vi "VMS_6_Controller.vi"() -> ()   [LabVIEW 2018]
uses:
  <vilib>/rvi/Emulation/niFpgaGetClockAttributes.vi
  <vilib>/rvi/Emulation/niFpgaSctlEmulationGetInTimedLoop.vi
  <vilib>/rvi/Emulation/niFpgaEmulationReportErrorSimple.vi
  <vilib>/rvi/Emulation/niFpgaProcessEmulError.vi
  <vilib>/rvi/eio/common/nirviEmuTemplateMethod_errors.vi
  <vilib>/rvi/Emulation/niFpgaCriticalErrorInLSC.vi
  <vilib>/rvi/interface/RandomDataEmulation/niFpgaRandomDataHandleErrors.vi
  <vilib>/rvi/occurrence/nirviWaitOnOccurrenceBase.vi
  <vilib>/eio/EIOMethodNode/EIOMethodNode.xnode
  <vilib>/rvi/DataTransferAndStorage/Container/XNode/niFpgaContainer.xnode
  <vilib>/rvi/interface/RandomDataEmulation/nirviRandomDataFpgaReadWriteTemplate.vi
  <vilib>/eio/EIONode/EIONode.xnode
panel:
  out "FIFO full":bool
  in  "Output type":i16
  in  "Period (ms)":u32=5
  out "Chassis Temperature":fxp<+/-,32,16>
  out "Stopped":bool
  out "Ready":bool
  out "Ticks":u64
  out "Timeouted":bool
  in  "Operate":bool
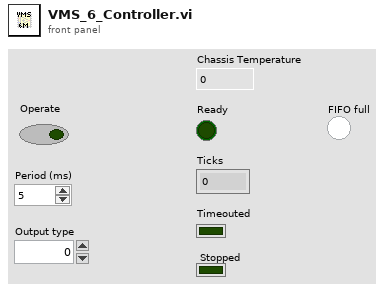
[diagram p1: front panel]
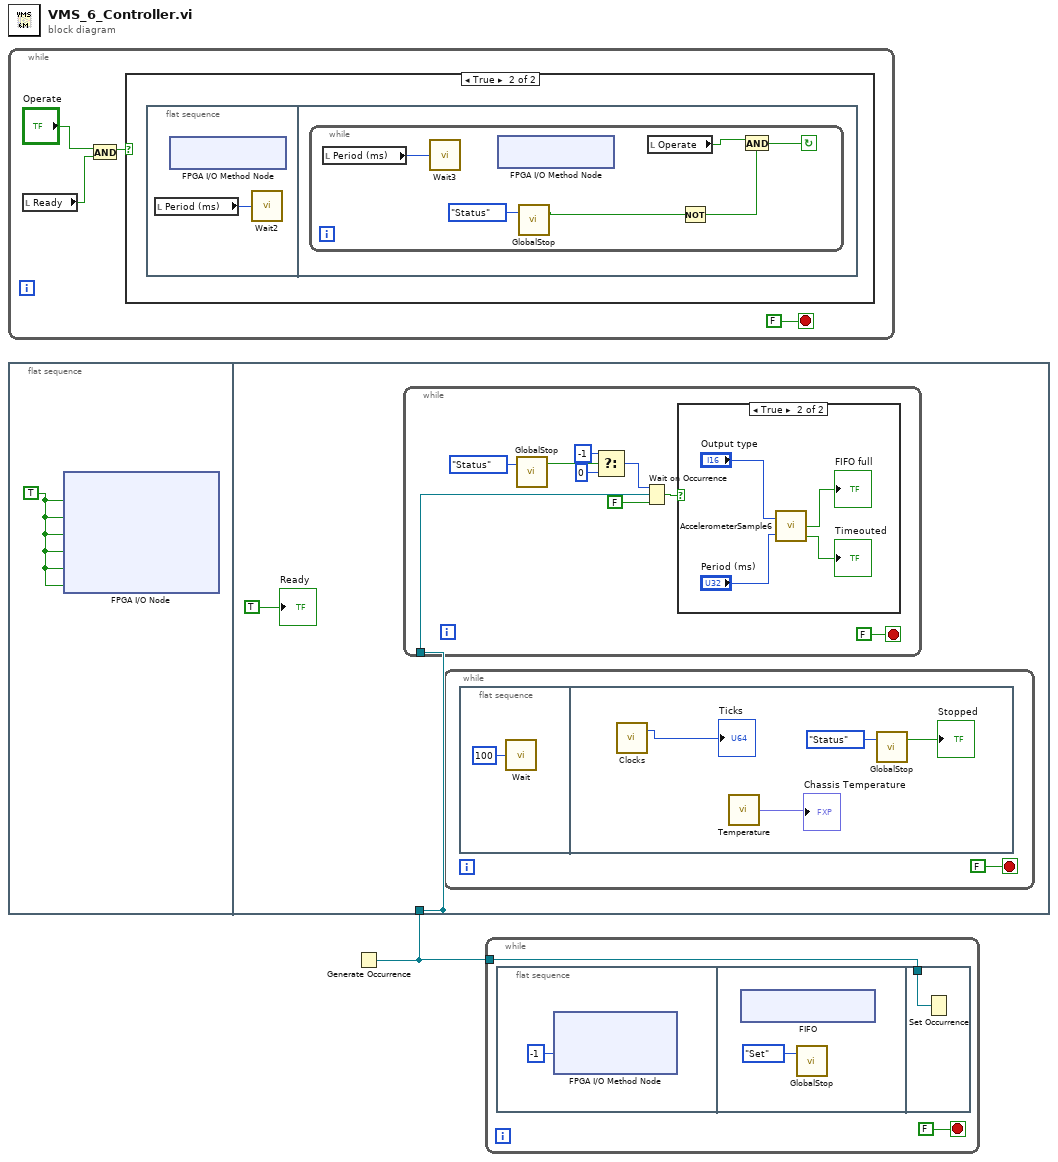
[diagram p0: block diagram]
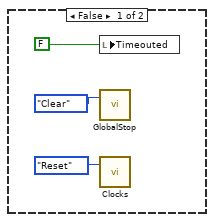
[diagram p2: hidden frame]
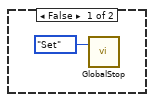
[diagram p3: hidden frame]
diagram:
  n1 = while {
    stop <- FALSE stop-if-true
    n2 = local read "Ready"() -> (w2:bool)
    n3 = And(x="Operate", y=w2) -> (x .and. y?=w4:bool)
    n4 = case shown="True" w4 {
      frame False {
        n5 = call "GlobalStop.vi"("Enum"=enum16{"Clear", "Set", "Status"}."Set") -> ()  [unwired: 1 in, 2 out]
      }
      frame True {
        n6 = flat-sequence {
          frame #0 {
            n7 = local read "Period (ms)"() -> (w7:u32)
            n8 = xnode "FPGA I/O Method Node"() -> ()  [unwired: 1 in, 1 out]
            n9 = call "Wait2"("Count(mSec)"=w7) -> ()  [unwired: 1 out]
          }
          frame #1 {
            n10 = while {
              stop <- w12 continue-if-true
              n11 = local read "Period (ms)"() -> (w8:u32)
              n12 = call "Wait3"("Count(mSec)"=w8) -> ()  [unwired: 1 out]
              n13 = xnode "FPGA I/O Method Node"() -> ()  [unwired: 1 in, 1 out]
              n14 = call "GlobalStop.vi"("Enum"=enum16{"Clear", "Set", "Status"}."Status") -> ("Boolean"=w9:bool)  [unwired: 1 in, 1 out]
              n15 = local read "Operate"() -> (w13:bool)
              n16 = Not(x=w9) -> (.not. x?=w11:bool)
              n17 = And(x=w13, y=w11) -> (x .and. y?=w12:bool)
            }
          }
        }
      }
    }
  }
  n18 = flat-sequence {
    tunnel: w1 -> [w15]
    tunnel: [w15] -> _
    frame #0 {
      w14 = TRUE ("Accelerometer5/Start")
      n19 = xnode "FPGA I/O Node"("Accelerometer1/Start"=w14, "Accelerometer2/Start"=w14, "Accelerometer3/Start"=w14, "Accelerometer4/Start"=w14, "Accelerometer5/Start"=w14, "Accelerometer6/Start"=w14) -> ()  [unwired: 6 in, 6 out]
    }
    frame #1 {
      n20 = while {
        tunnel: w15 -> [w28]
        stop <- FALSE stop-if-true
        n21 = call "GlobalStop.vi"("Enum"=enum16{"Clear", "Set", "Status"}."Status") -> ("Boolean"=w23:bool)  [unwired: 1 in, 1 out]
        n22 = Select(t=-1, s=w23, f=0) -> (s? t:f=w27:i32)
        n23 = Wait on Occurrence(1:FALSE ("ignore previous (T)"), 2:w28, 3:w27) -> (0:w29:bool)
        n24 = case shown="True" w29 {
          frame False {
            n25 = local write "Timeouted"(FALSE ("Timeouted")) -> ()
            n26 = call "GlobalStop.vi"("Enum"=enum16{"Clear", "Set", "Status"}."Clear") -> ()  [unwired: 1 in, 2 out]
            n27 = call "Clocks.vi"("Enum"=enum16{"Reset", "Increment", "Get"}."Reset") -> ()  [unwired: 1 in, 2 out]
          }
          frame True {
            n28 = call "AccelerometerSample6.vi"("Output type"="Output type", "Period (ms)"="Period (ms)") -> ("FIFO full"=→"FIFO full":bool, "Timeouted"=→"Timeouted":bool)  [unwired: 1 out]
          }
        }
      }
      n29 = while {
        stop <- FALSE stop-if-true
        n30 = flat-sequence {
          frame #0 {
            n31 = call "Wait"("Count(mSec)"=u32 100) -> ()  [unwired: 1 out]
          }
          frame #1 {
            n32 = call "Clocks.vi"() -> ("Clock"=→"Ticks":u64)  [unwired: 2 in, 1 out]
            n33 = call "Temperature.vi"() -> ("Mean temperature"=→"Chassis Temperature":fxp<+/-,32,16>)  [unwired: 1 in]
            n34 = call "GlobalStop.vi"("Enum"=enum16{"Clear", "Set", "Status"}."Status") -> ("Boolean"=→"Stopped":bool)  [unwired: 1 in, 1 out]
          }
        }
      }
      "Ready" <- TRUE ("Ready")
    }
  }
  n35 = Generate Occurrence() -> (w1:refnum<k4>)
  n36 = while {
    tunnel: w1 -> [w39]
    stop <- FALSE stop-if-true
    n37 = flat-sequence {
      tunnel: w39 -> [w43]
      frame #0 {
        n38 = xnode "FPGA I/O Method Node"("Timeout"=-1) -> ()  [unwired: 1 in, 2 out]
      }
      frame #1 {
        n39 = xnode "FIFO"() -> ()  [unwired: 1 in, 1 out]
        n40 = call "GlobalStop.vi"("Enum"=enum16{"Clear", "Set", "Status"}."Set") -> ()  [unwired: 1 in, 2 out]
      }
      frame #2 {
        n41 = Set Occurrence(w43) -> ()
      }
    }
  }
